vi "Format Log Results.vi"(8 "error in":errorcluster, 9 "Aperture Time":dbl[](array[numeric]), 10 "Source Mode":T1[](array[typedef]) items=["DC Voltage", "DC Current"], 11 "Pin Name":string[](array[string])) -> (0 "error out":errorcluster, 3 "Results":string[][](array[string]))   [LabVIEW 2024, in "devicePowerSequencerCoreLogic.lvlib"]
doc: "Formats Results . Adds PIn Name and Apperture time"
uses:
  devicePowerSequencerCoreLogic.lvlib
  controls/Source Mode.ctl
  Device Power Sequencer.lvlib
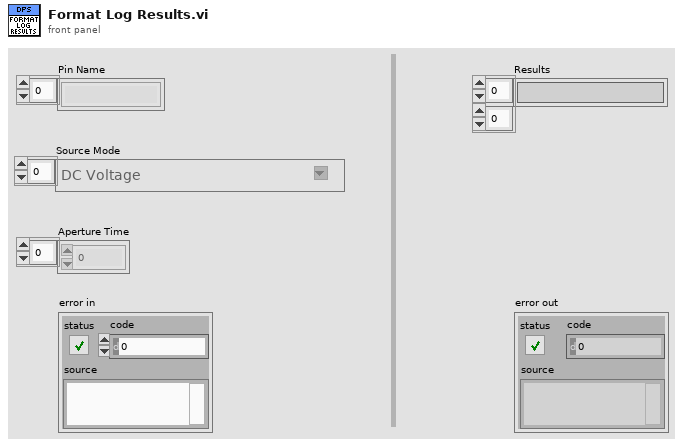
[diagram p1: front panel]
types:
  T1 = typedef "Device Power Sequencer.lvlib/Source Mode.ctl" = i32
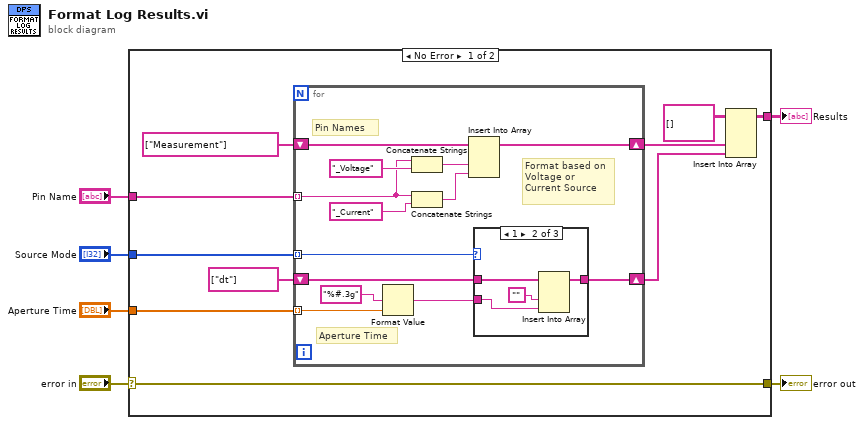
[diagram p0: block diagram]
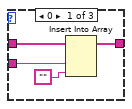
[diagram p2: hidden frame]
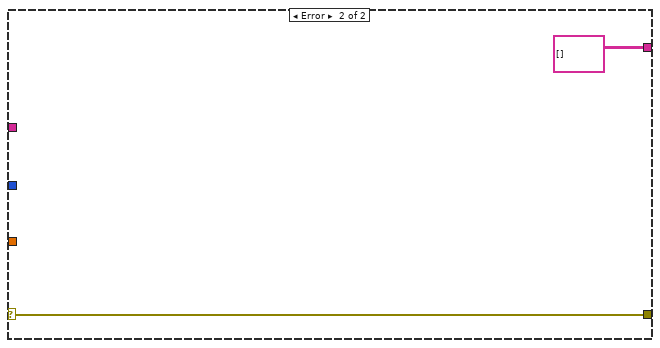
[diagram p4: hidden frame]
diagram:
  n1 = case shown="No Error" "error in" {
    selector: "error in" -> [w7 w39]
    tunnel: "Pin Name" -> [w13 _]
    tunnel: "Source Mode" -> [w12 _]
    tunnel: "Aperture Time" -> [w11 _]
    tunnel: [w8 string[][] [] ("element")] -> w4
    tunnel: [w7 w39] -> w3
    frame No Error {
      n2 = for {
        tunnel: w13 -> [w26] mode=indexing
        tunnel: w11 -> [w22] mode=indexing
        shift-right: [w19] -> w9
        shift-left: string[] ["dt"] -> [w20]
        tunnel: w12 -> [w18] mode=indexing
        shift-right: [w23] -> w10
        shift-left: string[] ["Measurement"] -> [w29]
        # "Aperture Time"
        # "Pin Names"
        # "Format based on Voltage or Current Source"
        n3 = Format Value(format string="%#.3g", value (0)=w22) -> (output string=w21:string)  [unwired: 1 in]
        n4 = Concatenate Strings(w26, "_Voltage" ("string")) -> (w28:string)
        n5 = Concatenate Strings(w26, "_Current" ("string")) -> (w24:string)
        n6 = Insert Into Array(array=w29, new element #1=w28, new element #2=w24) -> (w23:string[])  [unwired: 1 in]
        n7 = case shown="1" w18 {
          tunnel: w21 -> [w33 w34 _]
          tunnel: w20 -> [w32 w37 w38]
          tunnel: [w31 w36 w38] -> w19
          frame 0 {
            n8 = Insert Into Array(array=w32, new element #1=w33, new element #2="") -> (w31:string[])  [unwired: 1 in]
          }
          frame 1 {
            n9 = Insert Into Array(array=w37, new element #1="", new element #2=w34) -> (w36:string[])  [unwired: 1 in]
          }
          frame Default {
          }
        }
      }
      n10 = Insert Into Array(array=string[][] [] ("element"), new element #1=w10, new element #2=w9) -> (w8:string[][])  [unwired: 2 in]
    }
    frame Error {
    }
  }
  "Results" <- w4
  "error out" <- w3
